vi "Access File Compact Database.vi"(8 "error in":errorcluster caption="error in (no error)", 10 "Destination Access File Path":path caption="Destination Access File Path (*.mdb)", 11 "Source Access File Path":path caption="Source Access File Path (*.mdb)") -> (0 "error out":errorcluster, 3 "JRO.IJetEngine":refnum<k7>)   [LabVIEW 2014]
panel:
  in  "JRO.IJetEngine Local":refnum<k7>
  # "Input"
  # "Local"
  # "Output"
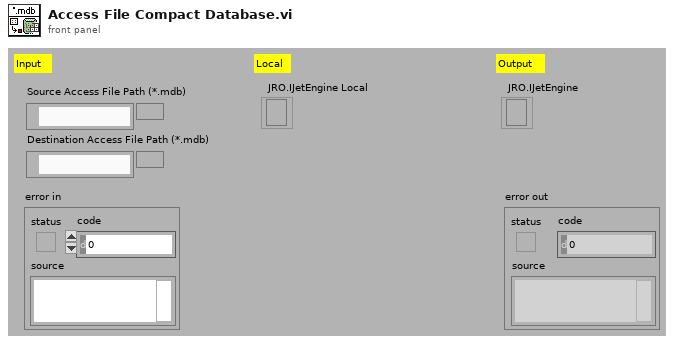
[diagram p1: front panel]
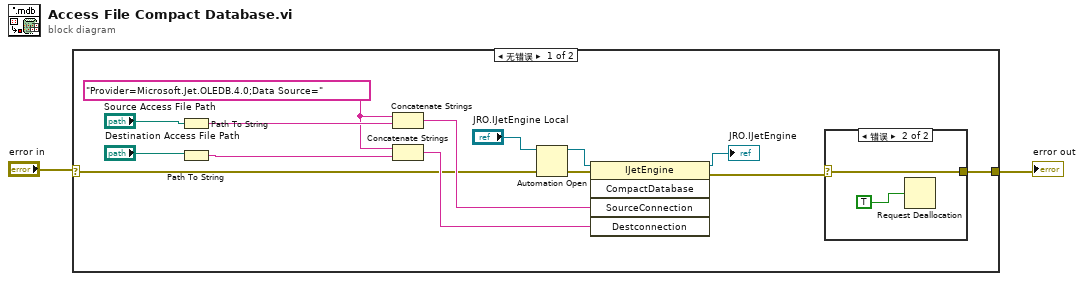
[diagram p0: block diagram]
diagram:
  n1 = case shown="无错误" "error in" {
    selector: "error in" -> [w8 w19]
    tunnel: [w5 w19] -> w1
    frame No Error {
      w12 = "Provider=Microsoft.Jet.OLEDB.4.0;Data Source="
      n2 = Path To String(path="Source Access File Path") -> (string=w13:string)
      n3 = Path To String(path="Destination Access File Path") -> (string=w11:string)
      n4 = Concatenate Strings(w12, w13) -> (w9:string)
      n5 = Concatenate Strings(w12, w11) -> (w10:string)
      n6 = Automation Open(Automation Refnum="JRO.IJetEngine Local") -> (Automation Refnum=w4:refnum<k7>)  [unwired: 3 in, 1 out]
      n7 = invoke class="IJetEngine" method="CompactDatabase"(reference=w4, error in=w8, "SourceConnection"=w9, "Destconnection"=w10) -> (reference out=→"JRO.IJetEngine":refnum<k7>, error out=w6:errorcluster)  [unwired: 1 in, 3 out]
      n8 = case shown="错误" w6 {
        selector: w6 -> [w16 w17]
        tunnel: [w16 w17] -> w5
        frame No Error {
        }
        frame Error {
          n9 = Request Deallocation(TRUE) -> ()
        }
      }
    }
    frame Error {
    }
  }
  "error out" <- w1
